vi "HEAVE UDP TRIAL 2.vi"() -> ()   [LabVIEW 2025]
panel:
  in  "min_finetune_floor":dbl=0.15
  in  "min_deadband_floor":dbl=0.05
  in  "Checkbox":bool
  in  "Fine Tune Zone":dbl=10.0
  out "Pulse delta":dbl
  in  "seconds to wait 3":dbl=1.0 format="%#_6p"
  in  "Max_pos_limit":dbl=50000000.0
  in  "Min_pos_limit":dbl
  in  "i_limit":dbl=10.0
  in  "Max Step Linit":dbl=10.0
  in  "Init Step":dbl=10.0
  in  "pct_scale":dbl=100.0
  in  "Deadband":dbl=0.1
  in  "Kd":dbl
  in  "Ki":dbl
  in  "Kp":dbl=1.0
  out "Current Position":dbl
  in  "Set Load":dbl
  in  "Current Load":dbl
  out "Node Id":u8
  in  "PID SPEED":sgl=80000.0
  in  "PID":bool
  in  "seconds to wait 2":dbl=0.2 format="%#_6p"
  out "Pulse Output":dbl
  out "Trigger":dbl
  in  "Low Command":dbl
  in  "High Command":dbl=10000.0
  in  "Time Low":dbl=1.5
  in  "Time High":dbl=1.5
  in  "dt":dbl=0.01
  out "fwMinor":u8
  out "fwMajor":u8
  out "faultCode":u16
  out "SURGE POSE":sgl format="%#.6f"
  out "HEAVE POSE":sgl format="%#.6f"
  out "Homed":u8
  out "State":u8
  out "Ack ID":u16
  in  "Write":bool
  in  "Read":bool
  in  "seconds to wait":dbl=0.001 format="%#_6p"
  in  "SPEED":sgl=10000.0
  in  "Distance":sgl=10000.0
  in  "Mode Command":u8=2
  out "Sequence ID":u16=7
  out "string 2":string
  in  "Stop Button":bool
  in  "Server Name":string="192.168.1.10"
  out "data out 2":string
  # "0100 0100 0000 0000 0000 0000 0000 00"
  # "0100 0100 0000 0000 0000 0000 0000 0000"
  # "100u"
  # "0500 0501 40C2 0C48 0000 0000 0000 0100"
  # "0300 0301 00CB E547 0000 0000 0000 0100"
  # "Home"
  # "0100 0100 0000 0000 0000 00"
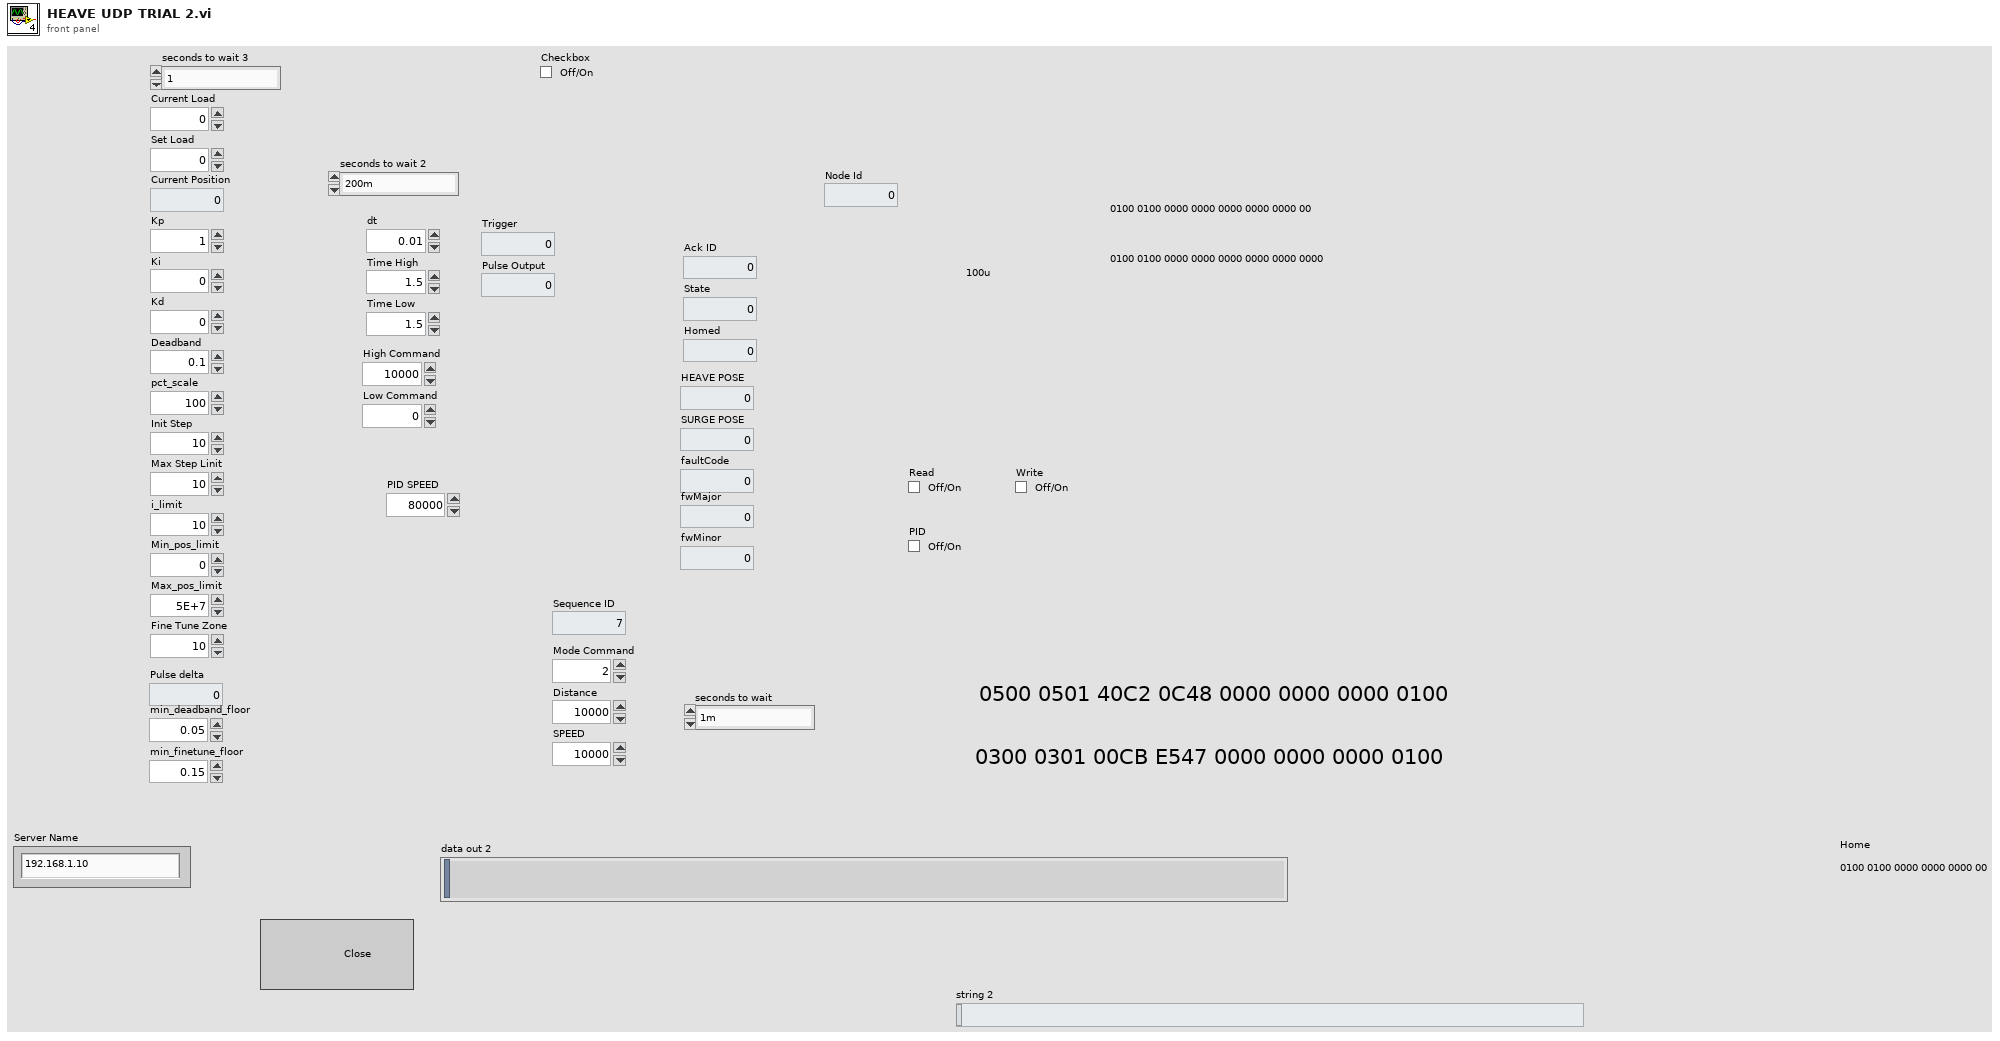
[diagram p1: front panel]
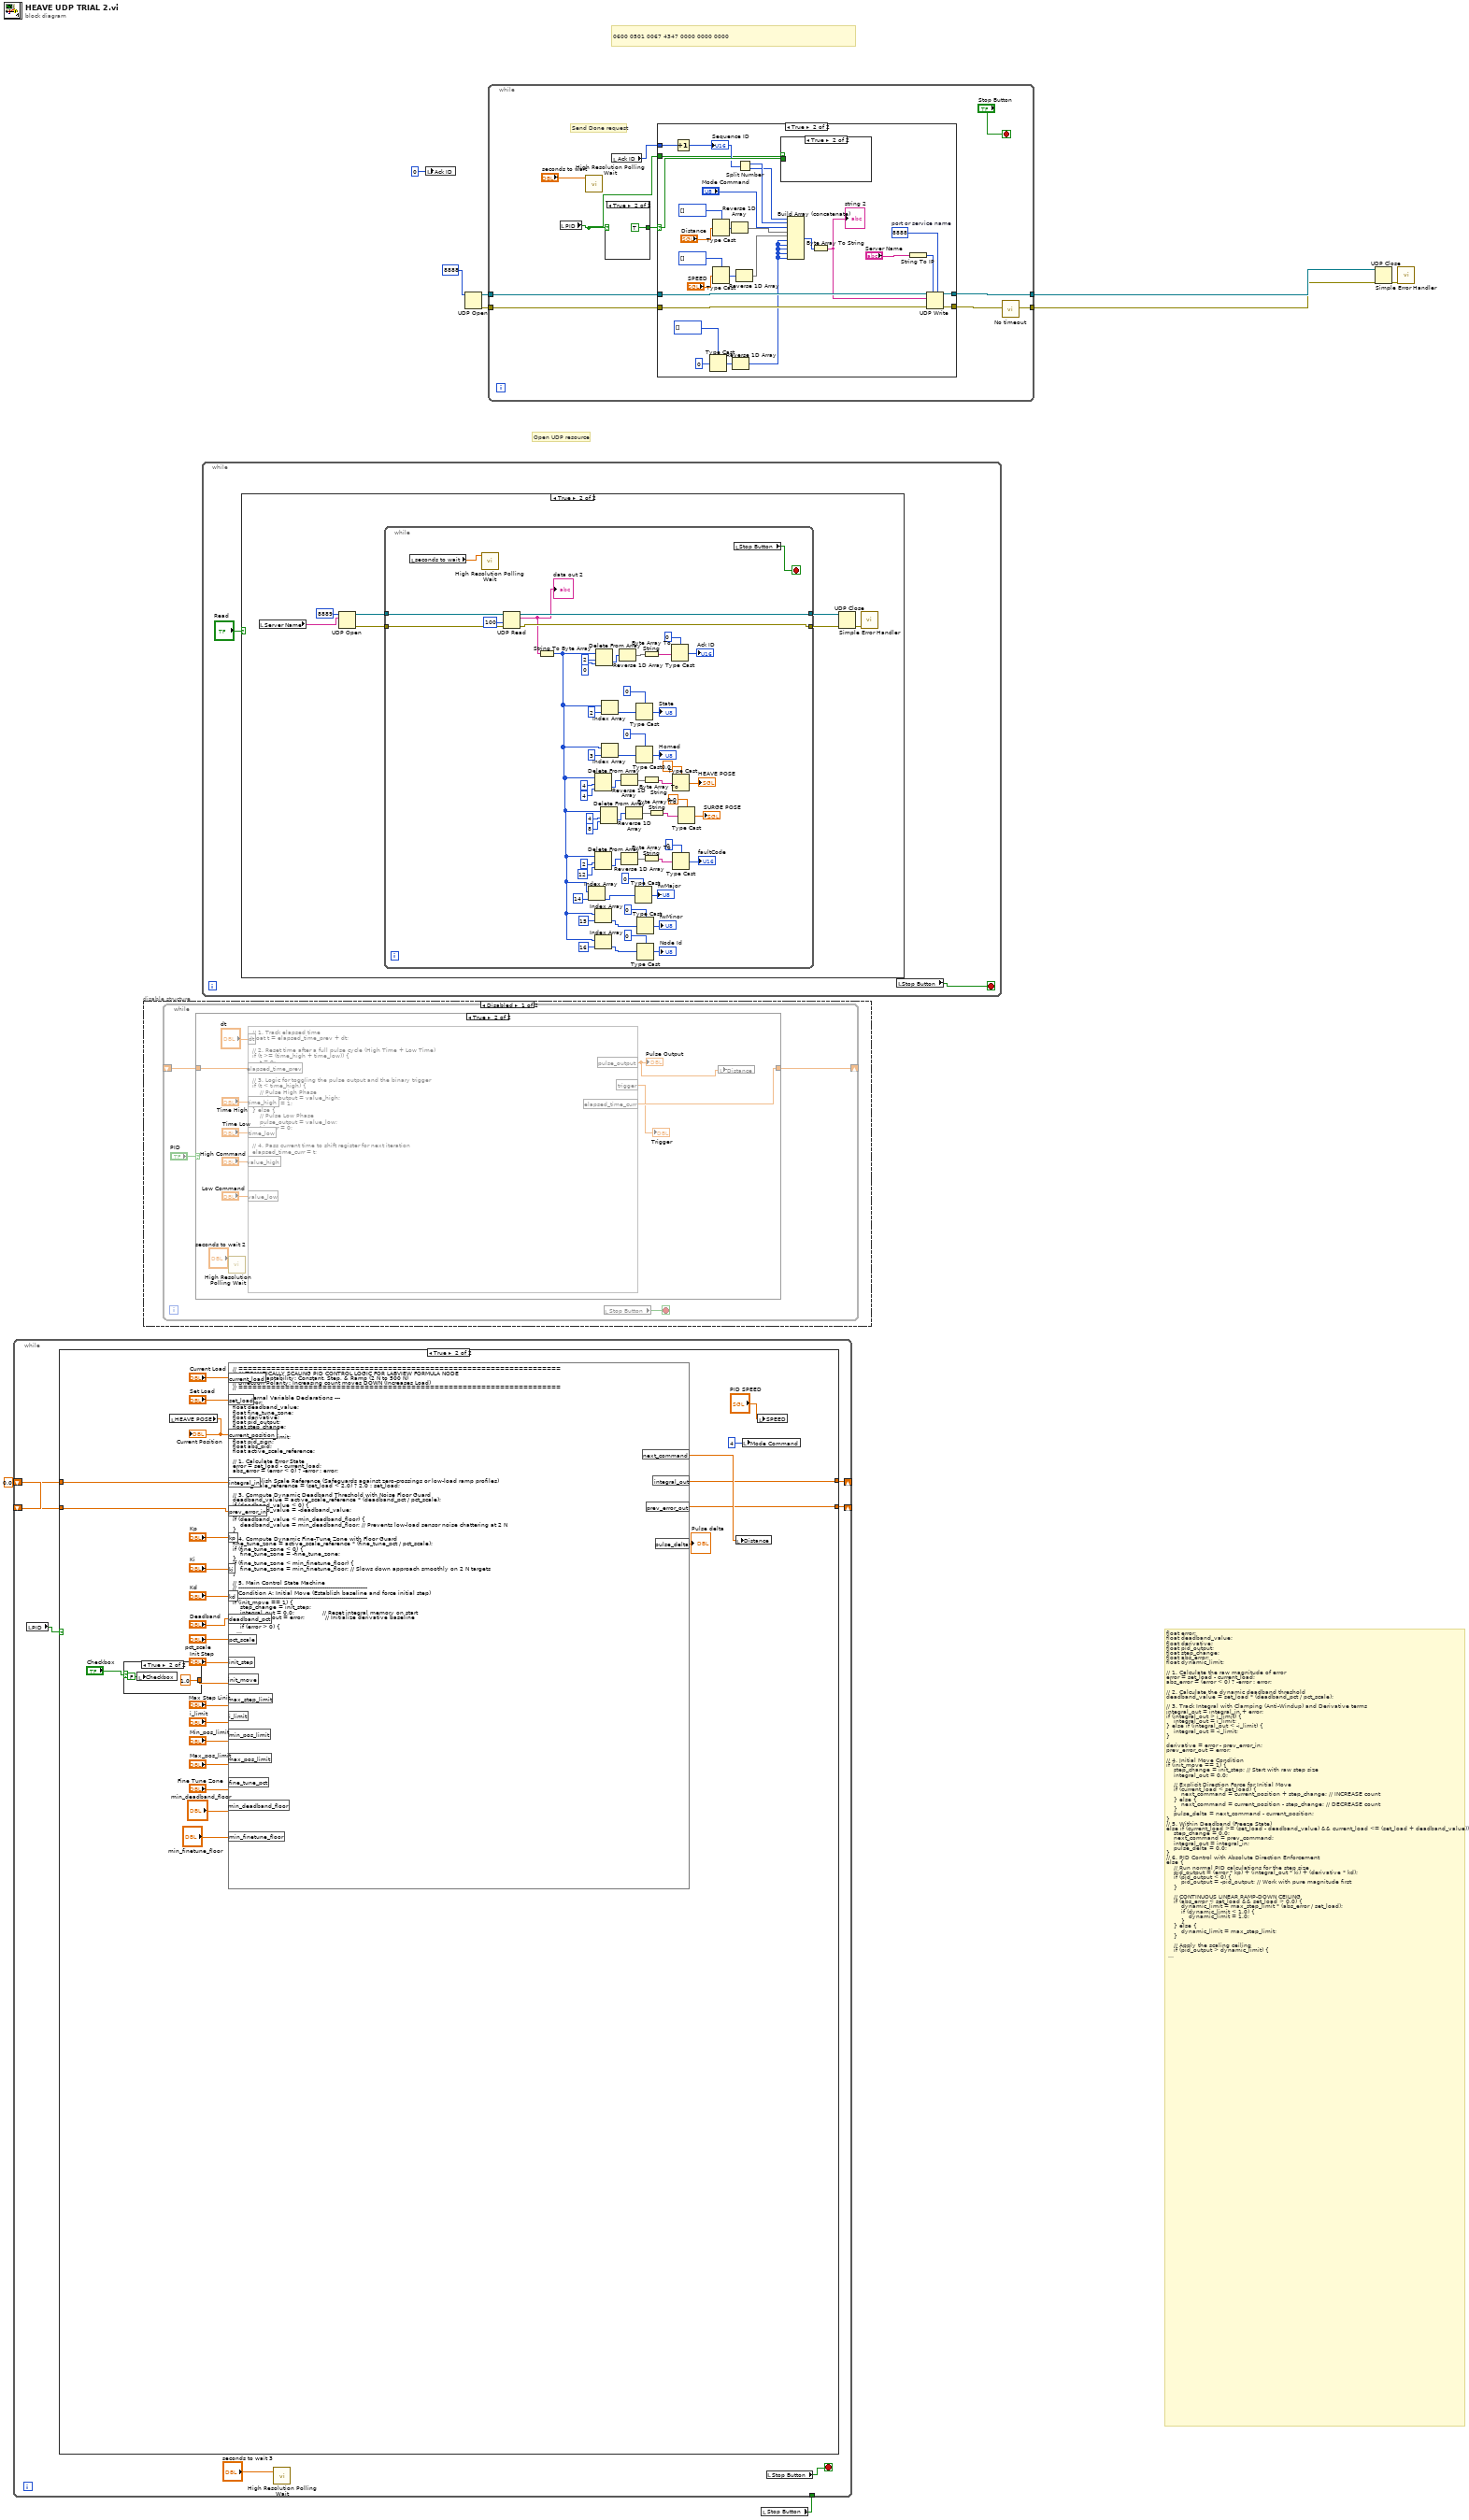
[diagram p0: block diagram]
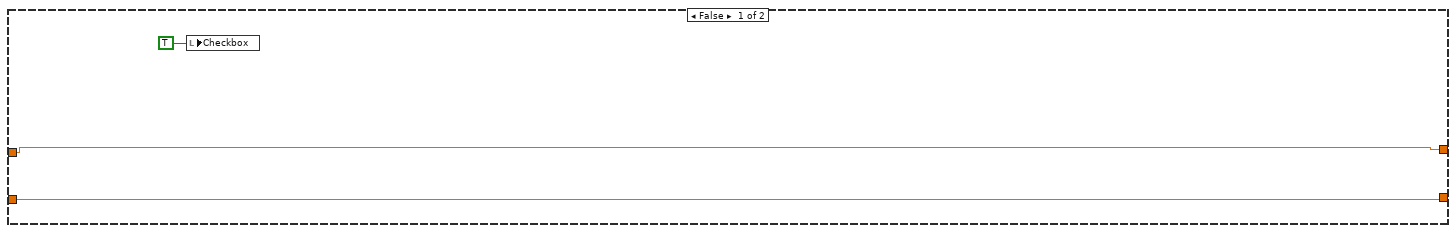
[diagram p2: hidden frame]
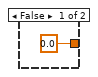
[diagram p3: hidden frame]
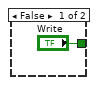
[diagram p7: hidden frame]
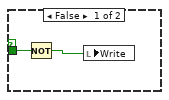
[diagram p9: hidden frame]
diagram:
  w1 = 0.0 ("integral_out")
  # "float error;\nfloat deadband_value;\nfloat derivative;\nfloat pid_output;\nfloat step_change;\nfloat abs_error;\nfloat dynamic_limit;\n\n// 1. Calculate the raw magnitude of error\nerror = set_load - current_load;\nabs_error = (error < 0) ? -error : error;\n\n// 2. Calculate the dynamic deadband threshold\ndeadband_value = set_load * (deadband_pct / pct_scale);\n\n// 3. Track Integral with Clamping (Anti-Windup) and Derivative terms\nintegral_out = integral_in + error;\nif (integral_out > i_limit) {\n    integral_out = i_limit;\n} else if (integral_out < -i_limit) {\n    integral_out = -i_limit;\n}\n\nderivative = error - prev_error_in;\nprev_error_out = error;\n\n// 4. Initial Move Condition\nif (init_move == 1) {\n    step_change = init_step; // Start with raw step size\n    integral_out = 0.0;\n    \n    // Explicit Direction Force for Initial Move\n    if (current_load < set_load) {\n        next_command = current_position + step_change; // INCREASE count\n    } else {\n        next_command = current_position - step_change; // DECREASE count\n    }\n    pulse_delta = next_command - current_position;\n}\n// 5. Within Deadband (Freeze State)\nelse if (current_load >= (set_load - deadband_value) && current_load <= (set_load + deadband_value)) {\n    step_change = 0.0;\n    next_command = prev_command;\n    integral_out = integral_in;\n    pulse_delta = 0.0;\n} \n// 6. PID Control with Absolute Direction Enforcement\nelse {\n    // Run normal PID calculations for the step size\n    pid_output = (error * kp) + (integral_out * ki) + (derivative * kd);\n    if (pid_output < 0) {\n        pid_output = -pid_output; // Work with pure magnitude first\n    }\n    \n    // CONTINUOUS LINEAR RAMP-DOWN CEILING\n    if (abs_error < set_load && set_load > 0.0) {\n        dynamic_limit = max_step_limit * (abs_error / set_load);\n        if (dynamic_limit < 1.0) {\n            dynamic_limit = 1.0;\n        }\n    } else {\n        dynamic_limit = max_step_limit;\n    }\n\n    // Apply the scaling ceiling\n    if (pid_output > dynamic_limit) {\n        step_change = dynamic_limit;\n    } else {\n        step_change = pid_output;\n    }\n    \n    // FORCED 1-COUNT PRECISION STEPPING BELOW THE THRESHOLD\n    if (abs_error <= fine_tune_zone) {\n        step_change = 1.0;\n    }\n\n    // -----------------------------------------------------------------\n    // CRITICAL FIX: ABSOLUTE DIRECTIONAL GUARANTEE\n    // -----------------------------------------------------------------\n    if (current_load < set_load) {\n        // Condition: Underloaded -> Motor count MUST increase\n        next_command = prev_command + step_change; \n    } else {\n        // Condition: Overloaded -> Motor count MUST decrease\n        next_command = prev_command - step_change; \n    }\n    \n    pulse_delta = next_command - prev_command;\n}\n\n// 7. Hard Absolute Safety Boundary Guard\nif (next_command > max_pos_limit) {\n    next_command = max_pos_limit;\n    pulse_delta = next_command - prev_command;\n} else if (next_command < min_pos_limit) {\n    next_command = min_pos_limit;\n    pulse_delta = next_command - prev_command;\n}"
  # "0600 0501 0067 4347 0000 0000 0000"
  # "Open UDP resource"
  n1 = disable-structure shown="Disabled" {
    frame Disabled {
      n2 = while {
        shift-right: [w11] -> _
        shift-left: _ -> [w12]
        stop <- w13 stop-if-true
        n3 = case shown="True" "PID" {
          tunnel: w12 -> [w14 w23]
          tunnel: [w14 w22] -> w11
          frame False {
          }
          frame True {
            n4 = call <vilib>:"High Resolution Polling Wait.vi"("seconds to wait"="seconds to wait 2") -> ()  [unwired: 10 in, 1 out]
            n5 = formula code="// 1. Track elapsed time\nfloat t = elapsed_time_prev + dt;\n\n// 2. Reset time after a full pulse cycle (High Time + Low Time)\nif (t >= (time_high + time_low)) {\n    t = 0;\n}\n\n// 3. Logic for toggling the pulse output and the binary trigger\nif (t < time_high) {\n    // Pulse High Phase\n    pulse_output = value_high;\n    trigger = 1; \n} else {\n    // Pulse Low Phase\n    pulse_output = value_low;\n    trigger = 0;\n}\n\n// 4. Pass current time to shift register for next iteration\nelapsed_time_curr = t;"("dt"="dt", "elapsed_time_prev"=w23, "time_high"="Time High", "time_low"="Time Low", "value_high"="High Command", "value_low"="Low Command") -> ("pulse_output"=w15:dbl, "trigger"=→"Trigger":dbl, "elapsed_time_curr"=w22:dbl)
            "Pulse Output" <- w15
            n6 = local write "Distance"(w15) -> ()
          }
        }
        n7 = local read "Stop Button"() -> (w13:bool)
      }
    }
    frame Enabled {
    }
  }
  n8 = while {
    stop <- w25 stop-if-true
    n9 = case shown="True" "Read" {
      frame False {
      }
      frame True {
        n10 = local read "Server Name"() -> (w30:string)
        n11 = UDP Open(10:w30, 11:u16 8889 ("port")) -> (port=w31:refnum<k16>, 0:w32:errorcluster)  [unwired: 3 in, 1 out]
        n12 = while {
          tunnel: w32 -> [w90]
          tunnel: w31 -> [w89]
          tunnel: [w88] -> w28
          tunnel: [w86] -> w27
          stop <- w87 stop-if-true
          n13 = local read "seconds to wait"() -> (w84:dbl)
          n14 = call <vilib>:"High Resolution Polling Wait.vi"("seconds to wait"=w84) -> ()  [unwired: 10 in, 1 out]
          n15 = UDP Read(connection ID=w89, timeout ms (25000)=100, 8:w90) -> (data out=w43:string, error out=w88:errorcluster, 3:w86:refnum<k16>)  [unwired: 1 in, 2 out]
          "data out 2" <- w43
          n16 = String To Byte Array(string=w43) -> (unsigned byte array=w34:u8[])
          n17 = Index Array(array=w34, index=14) -> (element=w47:u8)
          n18 = Delete From Array(array=w34, length=4, index=4) -> (deleted portion=w39:u8[])  [unwired: 1 out]
          n19 = Delete From Array(array=w34, length=2, index=12) -> (deleted portion=w40:u8[])  [unwired: 1 out]
          n20 = Index Array(array=w34, index=15) -> (element=w44:u8)
          n21 = Index Array(array=w34, index=16) -> (element=w38:u8)
          n22 = Delete From Array(array=w34, length=2, index=0) -> (deleted portion=w41:u8[])  [unwired: 1 out]
          n23 = Delete From Array(array=w34, length=4, index=8) -> (deleted portion=w42:u8[])  [unwired: 1 out]
          n24 = Index Array(array=w34, index=2) -> (element=w75:u8)
          n25 = Index Array(array=w34, index=3) -> (element=w72:u8)
          n26 = Reverse 1D Array(array=w41) -> (reversed array=w81:u8[])
          n27 = Reverse 1D Array(array=w39) -> (reversed array=w67:u8[])
          n28 = Reverse 1D Array(array=w40) -> (reversed array=w54:u8[])
          n29 = Reverse 1D Array(array=w42) -> (reversed array=w62:u8[])
          n30 = Type Cast(type=u8 0, x=w47) -> (*(type *) &x=→"fwMajor":u8)
          n31 = Type Cast(type=u8 0, x=w75) -> (*(type *) &x=→"State":u8)
          n32 = Type Cast(type=u8 0, x=w72) -> (*(type *) &x=→"Homed":u8)
          n33 = Type Cast(type=u8 0, x=w44) -> (*(type *) &x=→"fwMinor":u8)
          n34 = Type Cast(type=u8 0, x=w38) -> (*(type *) &x=→"Node Id":u8)
          n35 = Byte Array To String(unsigned byte array=w67) -> (string=w65:string)
          n36 = Byte Array To String(unsigned byte array=w54) -> (string=w53:string)
          n37 = Byte Array To String(unsigned byte array=w81) -> (string=w79:string)
          n38 = Byte Array To String(unsigned byte array=w62) -> (string=w63:string)
          n39 = Type Cast(type=u16 0, x=w79) -> (*(type *) &x=→"Ack ID":u16)
          n40 = Type Cast(type=sgl 0.0, x=w65) -> (*(type *) &x=→"HEAVE POSE":sgl)
          n41 = Type Cast(type=u16 0, x=w53) -> (*(type *) &x=→"faultCode":u16)
          n42 = Type Cast(type=sgl 0.0, x=w63) -> (*(type *) &x=→"SURGE POSE":sgl)
          n43 = local read "Stop Button"() -> (w87:bool)
        }
        n44 = UDP Close(connection ID=w27, 8:w28) -> (error out=w29:errorcluster)  [unwired: 1 out]
        n45 = call <vilib>:"Simple Error Handler.vi"("error in (no error)"=w29) -> ()  [unwired: 4 in, 5 out]
      }
    }
    n46 = local read "Stop Button"() -> (w25:bool)
  }
  n47 = local write "Ack ID"(u16 0 ("Ack ID")) -> ()
  n48 = UDP Open(11:u16 8888 ("port")) -> (port=w9:refnum<k16>, 0:w8:errorcluster)  [unwired: 4 in, 1 out]
  n49 = while {
    tunnel: w9 -> [w100]
    tunnel: w8 -> [w99]
    tunnel: [w97] -> w6
    tunnel: [w98] -> w5
    stop <- "Stop Button" stop-if-true
    # "Send Done request"
    n50 = local read "PID"() -> (w91:bool)
    n51 = call <vilib>:"High Resolution Polling Wait.vi"("seconds to wait"="seconds to wait") -> ()  [unwired: 10 in, 1 out]
    n52 = case shown="True" w91 {
      tunnel: ["Write" TRUE ("Write")] -> w93
      frame False {
      }
      frame True {
      }
    }
    n53 = local read "Ack ID"() -> (w92:u16)
    n54 = case shown="True" w93 {
      selector: w93 -> [_ w112]
      tunnel: w100 -> [w103 w132]
      tunnel: w99 -> [w104 w131]
      tunnel: [w103 w128] -> w97
      tunnel: [w104 w127] -> w96
      tunnel: w92 -> [_ w111]
      tunnel: w91 -> [_ w109]
      frame False {
      }
      frame True {
        w126 = u16 8888  # port or service name
        n55 = Increment(x=w111) -> (x+1=w110:u16)
        "Sequence ID" <- w110
        n56 = Type Cast(type=u8[] [], x=u8 0) -> (*(type *) &x=w108:u8[])
        n57 = Type Cast(type=u8[] [], x="Distance") -> (*(type *) &x=w119:u8[])
        n58 = Type Cast(type=u8[] [], x="SPEED") -> (*(type *) &x=w120:u8[])
        n59 = Reverse 1D Array(array=w119) -> (reversed array=w124:u8[])
        n60 = Reverse 1D Array(array=w108) -> (reversed array=w105:u8[])
        n61 = Reverse 1D Array(array=w120) -> (reversed array=w125:u8[])
        n62 = Split Number(x=w110) -> (hi(x)=w123:u8, lo(x)=w122:u8)
        n63 = case shown="True" w109 {
          tunnel: w112 -> [w134 _]
          frame False {
            n64 = Not(x=w134) -> (.not. x?=w133:bool)
            n65 = local write "Write"(w133) -> ()
          }
          frame True {
          }
        }
        n66 = Build Array (concatenate)(w122, w123, "Mode Command", w124, w125, w105, w105, w105, w105, w105) -> (w121:u8[])
        n67 = Byte Array To String(unsigned byte array=w121) -> (string=w115:string)
        "string 2" <- w115
        n68 = String To IP(1:"Server Name") -> (0:w129:u32)
        n69 = UDP Write(address=w129, port or service name=w126, connection ID=w132, data in=w115, 8:w131) -> (error out=w127:errorcluster, 3:w128:refnum<k16>)  [unwired: 1 in]
      }
    }
    n70 = call "No timeout.vi"("Error In"=w96) -> ("Error Out"=w98:errorcluster)  [unwired: 10 in]
  }
  n71 = local read "Stop Button"() -> (w2:bool)
  n72 = while {
    shift-right: [w140] -> _
    shift-left: w1 -> [w141]
    shift-right: [w138] -> _
    shift-left: w1 -> [w139]
    tunnel: w2 -> [_]
    stop <- w136 stop-if-true
    n73 = local read "PID"() -> (w135:bool)
    n74 = case shown="True" w135 {
      tunnel: w141 -> [w143 w169]
      tunnel: [w143 w168] -> w140
      tunnel: w139 -> [w144 w167]
      tunnel: [w144 w166] -> w138
      frame False {
        n75 = local write "Checkbox"(TRUE ("Checkbox")) -> ()
      }
      frame True {
        n76 = case shown="True" "Checkbox" {
          tunnel: [0.0 ("Init Move") 1.0 ("Init Move")] -> w157
          frame False {
          }
          frame True {
            n77 = local write "Checkbox"(FALSE ("Checkbox")) -> ()
          }
        }
        n78 = local read "HEAVE POSE"() -> (w152:sgl)
        "Current Position" <- w152
        n79 = formula code="// =====================================================================\n// AUTOMATICALLY SCALING PID CONTROL LOGIC FOR LABVIEW FORMULA NODE\n// Profile Adaptability: Constant, Step, & Ramp (2 N to 500 N)\n// Direction Polarity: Increasing count moves DOWN (Increases Load)\n// =====================================================================\n\n// --- Internal Variable Declarations ---\nfloat error;\nfloat deadband_value;\nfloat fine_tune_zone;\nfloat derivative;\nfloat pid_output;\nfloat step_change;\nfloat abs_error;\nfloat dynamic_limit;\nfloat pid_sign;\nfloat abs_pid;\nfloat active_scale_reference;\n\n// 1. Calculate Error State\nerror = set_load - current_load;\nabs_error = (error < 0) ? -error : error;\n\n// 2. Establish Scale Reference (Safeguards against zero-crossings or low-load ramp profiles)\nactive_scale_reference = (set_load < 2.0) ? 2.0 : set_load;\n\n// 3. Compute Dynamic Deadband Threshold with Noise Floor Guard\ndeadband_value = active_scale_reference * (deadband_pct / pct_scale);\nif (deadband_value < 0) {\n    deadband_value = -deadband_value; \n}\nif (deadband_value < min_deadband_floor) {\n    deadband_value = min_deadband_floor; // Prevents low-load sensor noise chattering at 2 N\n}\n\n// 4. Compute Dynamic Fine-Tune Zone with Floor Guard\nfine_tune_zone = active_scale_reference * (fine_tune_pct / pct_scale);\nif (fine_tune_zone < 0) {\n    fine_tune_zone = -fine_tune_zone;\n}\nif (fine_tune_zone < min_finetune_floor) {\n    fine_tune_zone = min_finetune_floor; // Slows down approach smoothly on 2 N targets\n}\n\n// 5. Main Control State Machine\n// ---------------------------------------------------------------------\n// Condition A: Initial Move (Establish baseline and force initial step)\n// ---------------------------------------------------------------------\nif (init_move == 1) {\n    step_change = init_step; \n    integral_out = 0.0;               // Reset integral memory on start\n    prev_error_out = error;           // Initialize derivative baseline\n    \n    if (error > 0) {\n        next_command = current_position + step_change;\n    } else {\n        next_command = current_position - step_change;\n    }\n    pulse_delta = next_command - current_position;\n}\n// ---------------------------------------------------------------------\n// Condition B: Within Target Deadband (Freeze State / Zero Energy)\n// ---------------------------------------------------------------------\nelse if (abs_error <= deadband_value) {\n    step_change = 0.0;\n    next_command = current_position; // Lock to current physical position\n    integral_out = integral_in;       // Freeze integral to prevent drift\n    prev_error_out = error;           // Keep derivative baseline fresh\n    pulse_delta = 0.0;\n} \n// ---------------------------------------------------------------------\n// Condition C: Active PID Control Zone\n// ---------------------------------------------------------------------\nelse {\n    // A. Track Integral with strict Anti-Windup Limits\n    integral_out = integral_in + error;\n    if (integral_out > i_limit) {\n        integral_out = i_limit;\n    } else if (integral_out < -i_limit) {\n        integral_out = -i_limit;\n    }\n\n    // B. Calculate Derivative (Tracks rate of change of error - crucial for RAMP tracking)\n    derivative = error - prev_error_in;\n    prev_error_out = error; \n\n    // C. Execute Raw PID Equation\n    pid_output = (error * kp) + (integral_out * ki) + (derivative * kd);\n    \n    // D. Extract Mathematical Sign and Magnitude\n    pid_sign = (pid_output >= 0) ? 1.0 : -1.0;\n    abs_pid = (pid_output < 0) ? -pid_output : pid_output;\n\n    // E. Continuous Linear Ramp-Down Ceiling (Smooth adaptation for moving ramp profiles)\n    if (abs_error < active_scale_reference) {\n        dynamic_limit = max_step_limit * (abs_error / active_scale_reference);\n        if (dynamic_limit < 1.0) {\n            dynamic_limit = 1.0; // Minimum microstep velocity floor\n        }\n    } else {\n        dynamic_limit = max_step_limit; // Maximum speed deployment for STEP jumps\n    }\n\n    // F. Apply Smooth Step Control & Fine Tuning Zone\n    if (abs_error <= fine_tune_zone) {\n        step_change = 1.0; // Forced 1-Count Precision micro-stepping close to target\n    } else {\n        if (abs_pid < dynamic_limit) {\n            step_change = abs_pid; // Decay step size perfectly near steady state\n        } else {\n            step_change = dynamic_limit; // Cap velocity ceiling to prevent overshooting\n        }\n    }\n    \n    // G. Apply Step Vector directly relative to physical position\n    next_command = current_position + (step_change * pid_sign);\n    pulse_delta = next_command - current_position;\n}\n\n// 6. Hard Structural Boundaries & Safety Guards\n// ---------------------------------------------------------------------\nif (next_command > max_pos_limit) {\n    next_command = max_pos_limit;\n    pulse_delta = next_command - current_position;\n} else if (next_command < min_pos_limit) {\n    next_command = min_pos_limit;\n    pulse_delta = next_command - current_position;\n}"("current_load"="Current Load", "set_load"="Set Load", "current_position"=w152, "integral_in"=w169, "prev_error_in"=w167, "kp"="Kp", "ki"="Ki", "kd"="Kd", "deadband_pct"="Deadband", "pct_scale"="pct_scale", "init_step"="Init Step", "init_move"=w157, "max_step_limit"="Max Step Linit", "i_limit"="i_limit", "min_pos_limit"="Min_pos_limit", "max_pos_limit"="Max_pos_limit", "fine_tune_pct"="Fine Tune Zone", "min_deadband_floor"="min_deadband_floor", "min_finetune_floor"="min_finetune_floor") -> ("next_command"=w170:dbl, "integral_out"=w168:dbl, "prev_error_out"=w166:dbl, "pulse_delta"=→"Pulse delta":dbl)
        n80 = local write "Distance"(w170) -> ()
        n81 = local write "Mode Command"(u8 4 ("Mode Command")) -> ()
        n82 = local write "SPEED"("PID SPEED") -> ()
      }
    }
    n83 = call <vilib>:"High Resolution Polling Wait.vi"("seconds to wait"="seconds to wait 3") -> ()  [unwired: 10 in, 1 out]
    n84 = local read "Stop Button"() -> (w136:bool)
  }
  n85 = UDP Close(connection ID=w6, 8:w5) -> (error out=w4:errorcluster)  [unwired: 1 out]
  n86 = call <vilib>:"Simple Error Handler.vi"("error in (no error)"=w4) -> ()  [unwired: 4 in, 5 out]
